vi "Event_Structures.vi"() -> ()   [LabVIEW 2017]
panel:
  out "String 2":string
  in  "RESET":bool
  in  "stop":bool
  in  "String":string="Change me."
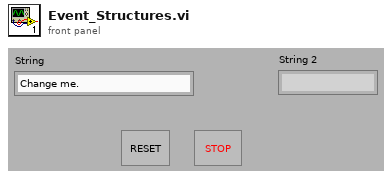
[diagram p1: front panel]
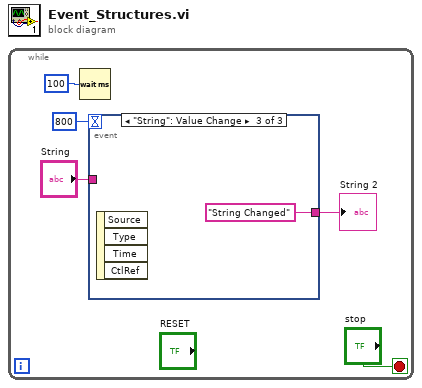
[diagram p0: block diagram]
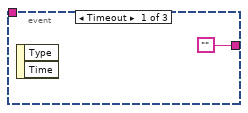
[diagram p2: hidden frame]
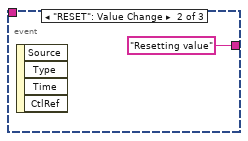
[diagram p3: hidden frame]
diagram:
  n1 = while {
    stop <- "stop" stop-if-true
    n2 = Wait (ms)(milliseconds to wait=u32 100) -> ()  [unwired: 1 out]
    n3 = event shown="[2] \"String\": Value Change" {
      selector: _ -> [_ _ _]
      dyn-events: _ -> [_ _ _]
      timeout: 800 -> [_ _ _]
      tunnel: ["" "Resetting value" "String Changed"] -> w2
      tunnel: "String" -> [_ _ _]
      event Timeout {
        n4 = event-data() -> ()  [unwired: 1 in, 2 out]
      }
      event "RESET": Value Change {
        n5 = event-data() -> ()  [unwired: 1 in, 4 out]
      }
      event "String": Value Change {
        n6 = event-data() -> ()  [unwired: 1 in, 4 out]
      }
    }
    "String 2" <- w2
  }
